vi "Handle Duplicate State Change.vi"(8 "error in (no error)":errorcluster, 9 "State":string, 11 "Routing Channel Ref in":T1 format="%.0x") -> (0 "error out":errorcluster, 1 "New State Added":string, 3 "Routing Channel Ref out":T1 format="%.0x")   [LabVIEW 2017, in "Routing and Faulting System Explorer.lvlib"]
uses:
  Routing and Faulting System Explorer.lvlib
  <vilib>/NI Veristand/Custom Device API/Custom Device Item Ref.ctl
  Scripting/Routing and Faulting Scripting.lvlib
  <vilib>/NI VeriStand/Custom Device API/Custom Device API.lvlib
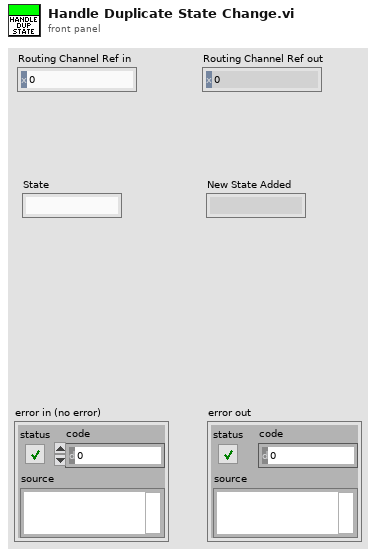
[diagram p1: front panel]
types:
  T1 = typedef "Custom Device API.lvlib/Custom Device Item Ref.ctl" = u64
  T2 = typedef "Routing and Faulting Shared.lvlib/Routing State.ctl" = cluster{"Name":string, "Description":string, "Value":i32, "Connection List":T3[]}
  T3 = typedef "Routing and Faulting Shared.lvlib/Connection.ctl" = cluster{"Resource":string, "Source":string, "Destination":string}
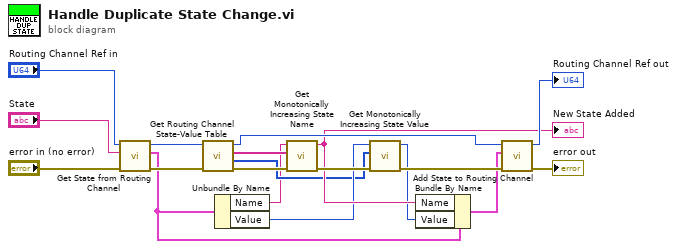
[diagram p0: block diagram]
diagram:
  n1 = call "Get State from Routing Channel.vi"("error in (no error)"="error in (no error)", "State"="State", "Channel Ref in"="Routing Channel Ref in") -> ("error out"=w15:errorcluster, "State and Connections"=w9:T2, "Channel Ref out"=w16:T1)  [unwired: 6 in]
  n2 = call "Get Routing Channel State-Value Table.vi"("error in (no error)"=w15, "Channel Ref in"=w16) -> ("error out"=w14:errorcluster, "State Values"=w3:i32[], "State Names"=w2:string[], "Channel Ref out"=w11:T1)  [unwired: 6 in]
  n3 = Unbundle By Name(w9) -> ("Name"=w1:string, "Value"=w4:i32)
  n4 = call "Get Monotonically Increasing State Name.vi"("error in (no error)"=w14, "State Names"=w2, "Desired State Name"=w1) -> ("error out"=w17:errorcluster, "New State Name"=w6:string)  [unwired: 7 in]
  "New State Added" <- w6
  n5 = call "Get Monotonically Increasing State Value.vi"("error in (no error)"=w17, "State Values"=w3, "Desire State Value"=w4) -> ("error out"=w13:errorcluster, "New State Value"=w5:i32)  [unwired: 7 in]
  n6 = Bundle By Name(cluster=w9, "Name"=w6, "Value"=w5) -> (w8:T2)
  n7 = call "Add State to Routing Channel.vi"("error in (no error)"=w13, "State and Connections"=w8, "Channel Ref in"=w11) -> ("error out"=→"error out":errorcluster, "Channel Ref out"=→"Routing Channel Ref out":T1)  [unwired: 7 in]
